vi "24_16_matrix_vector_multiply.vi"(3 "n":i32, 4 "m":i32, 5 "B":fxp<+/-,24,16>[](array[numeric]), 6 "A":fxp<+/-,24,16>[](array[numeric])) -> (0 "C":fxp<+/-,24,16>[](array[numeric]))   [LabVIEW 2020]
panel:
  in  "accum":fxp<+/-,24,16>
  in  "C_type":fxp<+/-,24,16>
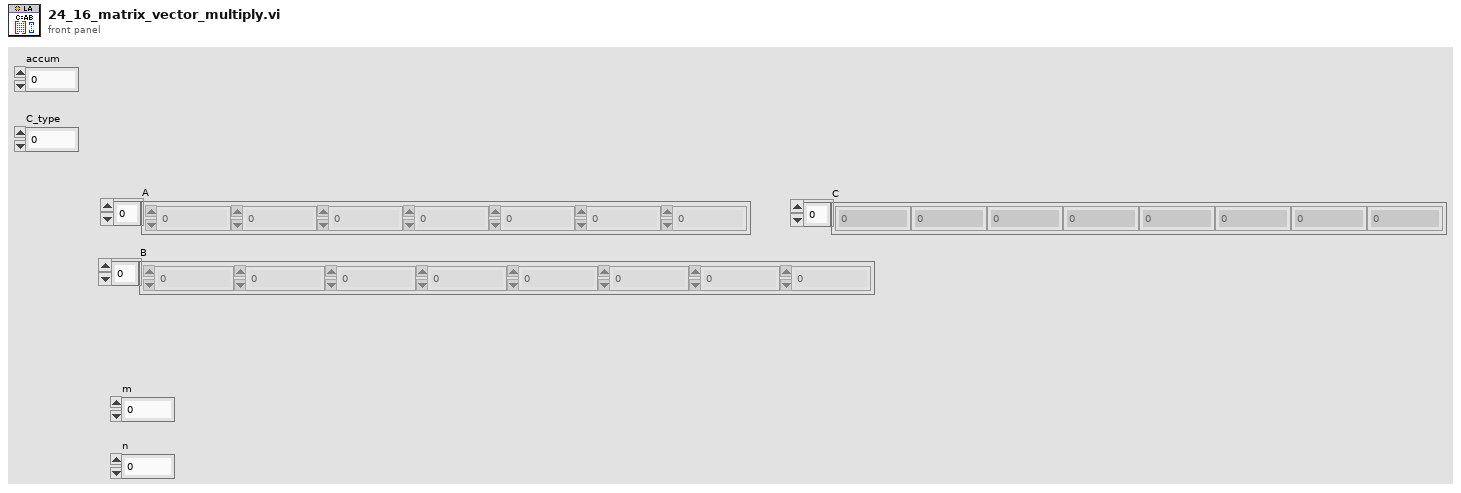
[diagram p1: front panel]
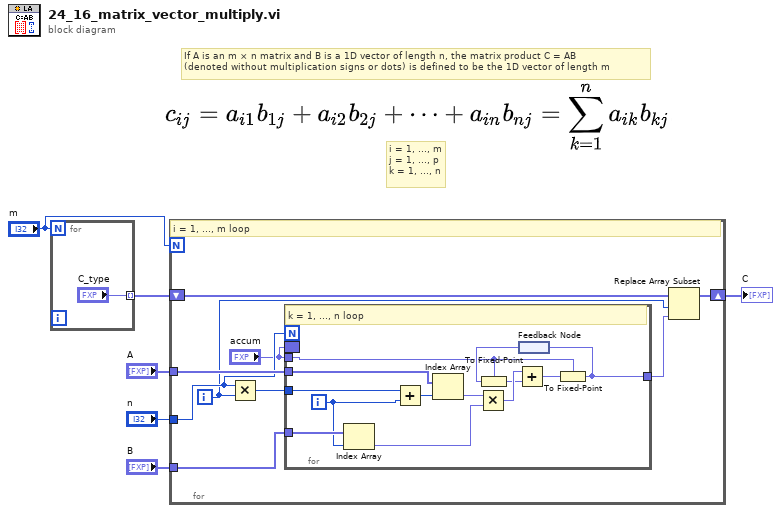
[diagram p0: block diagram]
diagram:
  # "If A is an m × n matrix and B is a 1D vector of length n, the matrix product C = AB \n(denoted without multiplication signs or dots) is defined to be the 1D vector of length m"
  # "i = 1, ..., m\nj = 1, ..., p\nk = 1, ..., n"
  n1 = for {
    N: "m" -> [_]
    tunnel: ["C_type"] -> w2 mode=indexing
  }
  n2 = for {
    N: "m" -> [_]
    tunnel: "B" -> [w16]
    tunnel: "A" -> [w13]
    tunnel: "n" -> [w12]
    shift-right: [w14] -> w4
    shift-left: w2 -> [w15]
    i -> [w9]
    # "i = 1, ..., m loop"
    n3 = Multiply(x=w12, y=w9) -> (x*y=w10:i32)
    n4 = for {
      N: w12 -> [_]
      tunnel: w13 -> [w29]
      tunnel: w10 -> [w23]
      tunnel: w16 -> [w28]
      tunnel: [w20] -> w11
      border: "accum" -> [_]
      tunnel: "accum" -> [w17]
      i -> [w22]
      # "k = 1, ..., n loop"
      n5 = Index Array(array=w28, index=w22) -> (element=w26:fxp<+/-,24,16>)
      n6 = Add(x=w23, y=w22) -> (x+y=w24:i32)
      n7 = Index Array(array=w29, index=w24) -> (element=w27:fxp<+/-,24,16>)
      n8 = Multiply(x=w27, y=w26) -> (x*y=w25:fxp<+/-,48,32>)
      n9 = feedback #1() -> (w18:fxp<+/-,24,16>)
      n10 = To Fixed-Point(fixed-point type=w17, number=w18) -> (fixed-point=w19:fxp<+/-,24,16>)
      n11 = Add(x=w25, y=w19) -> (x+y=w21:fxp<+/-,48,32>)
      n12 = To Fixed-Point(fixed-point type=w17, number=w21) -> (fixed-point=w20:fxp<+/-,24,16>)
      n13 = feedback-in #1(w20) -> ()
    }
    n14 = Replace Array Subset(array=w15, new element=w11, index=w9) -> (w14:fxp<+/-,24,16>[])
  }
  "C" <- w4
